vi "Get DB Record.vi"(8 "error in (no error)":errorcluster, 10 "Record":T1 {"Balance" format="%.2f"}, 11 "ATM Controller in":refnum<class "ATM Controller.lvclass">) -> (0 "error out":errorcluster, 3 "ATM Controller out":refnum<class "ATM Controller.lvclass">)   [LabVIEW 2019, in "ATM Controller.lvlib" / "ATM Controller.lvclass"]
uses:
  ATM Controller.lvclass
  Configuration Database/Configuration Database/Record -Cluster.ctl
  ATM Controller.lvclass/ATM Controller.ctl
  Configuration Database/Configuration Database/Configuration Database.lvclass
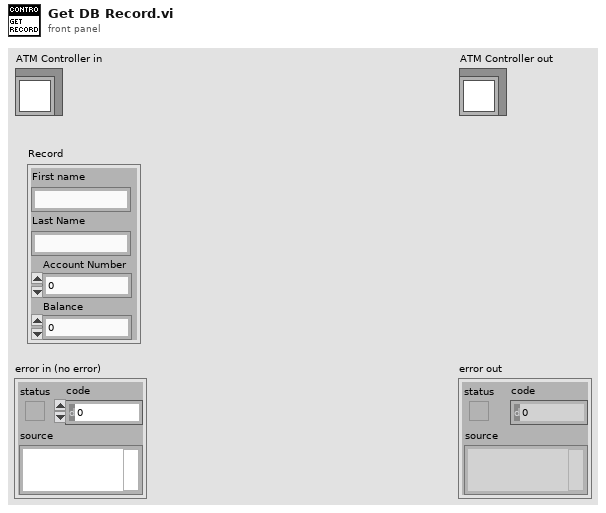
[diagram p1: front panel]
types:
  T1 = typedef "Configuration Database.lvlib/Configuration Database.lvclass/Record -Cluster.ctl" = cluster{"First name":string, "Last Name":string, "Account Number":u16, "Balance":u32}
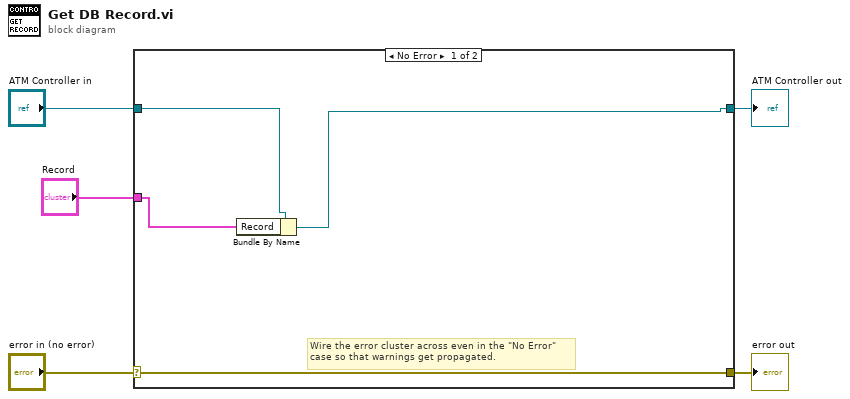
[diagram p0: block diagram]
diagram:
  n1 = case shown="No Error" "error in (no error)" {
    selector: "error in (no error)" -> [w9 w11]
    tunnel: [w9 w11] -> w4
    tunnel: [w6 w10] -> w2
    tunnel: "ATM Controller in" -> [w8 w10]
    tunnel: "Record" -> [w7 _]
    frame No Error {
      # "Wire the error cluster across even in the \"No Error\"\ncase so that warnings get propagated."
      n2 = Bundle By Name(cluster=w8, "Record"=w7) -> (w6:refnum<class "ATM Controller.lvclass">)
    }
    frame Error {
    }
  }
  "error out" <- w4
  "ATM Controller out" <- w2
